vi "microFPGA_laser_sequence_addr_20_ctrl.vi"(0 "VISA resource name":refnum<visa-resource-name>, 1 "laser channel":u16(ring)=3 items=["channel No 0", "channel No 1", "channel No 2", "channel No 3", "channel No 4", "channel No 5", "channel No 6"], 2 "write or read":u16(ring) items=["read", "write"], 5 "sequence write":bool[](array[boolean])=[FALSE, FALSE, FALSE, FALSE, FALSE, FALSE, FALSE, FALSE, FALSE, FALSE, FALSE, FALSE, FALSE, FALSE, FALSE, FALSE], 11 "error in (no error)":errorcluster) -> (4 "VISA resource name 2":refnum<visa-resource-name>, 6 "sequence read":bool[](array[boolean]), 8 "value write confirm":bool, 10 "abort_wrong_input":bool, 15 "error out":errorcluster)   [LabVIEW 2016]
panel:
  out "mode read string answer":string
  out "mode read string":string
  out "mode write string":string
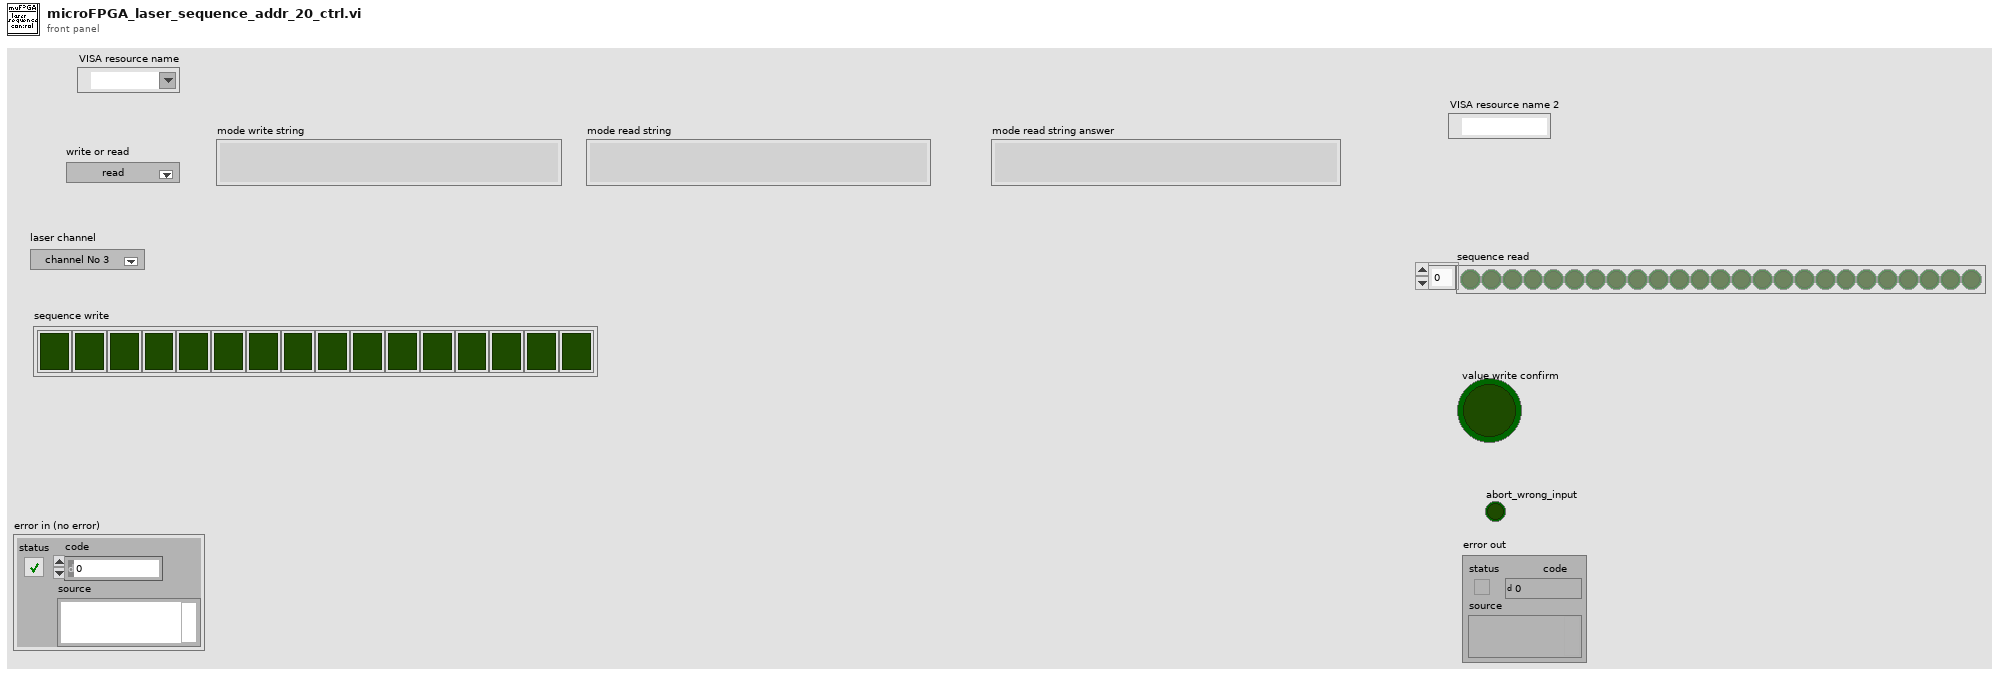
[diagram p1: front panel]
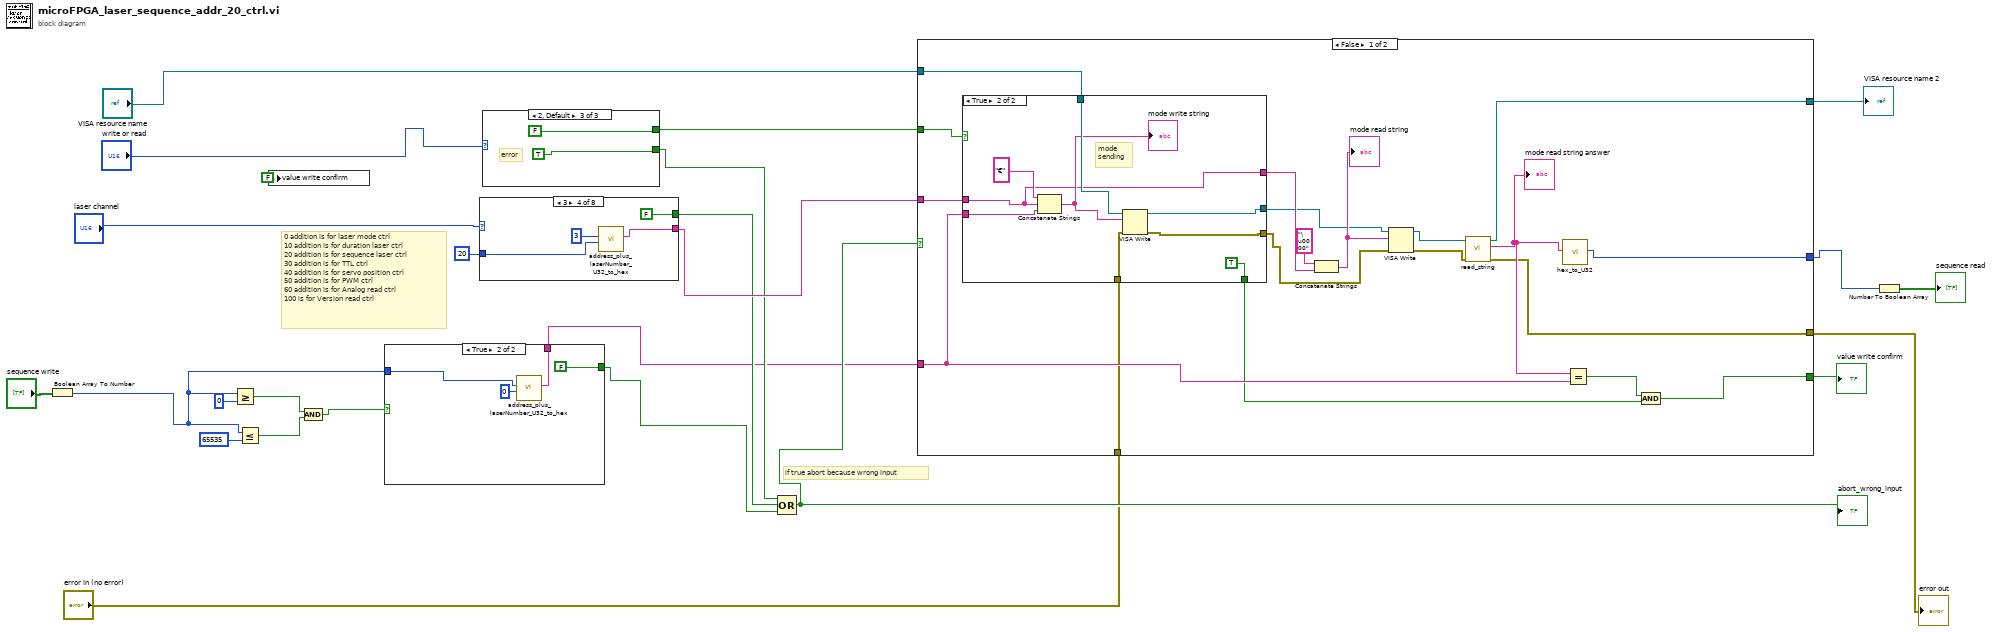
[diagram p0: block diagram]
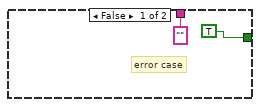
[diagram p2: hidden frame]
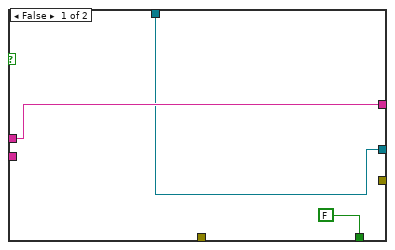
[diagram p3: hidden frame]
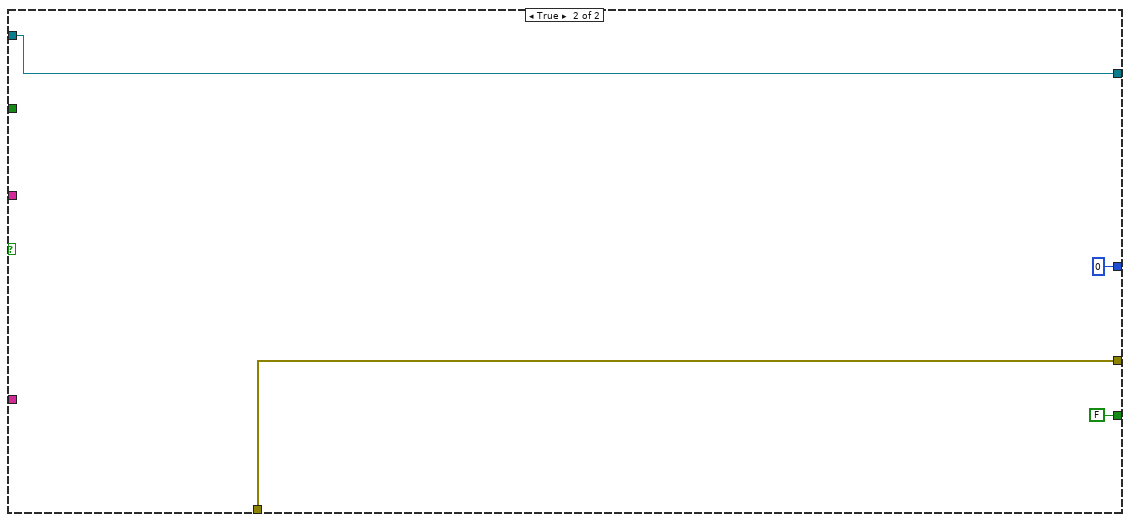
[diagram p4: hidden frame]
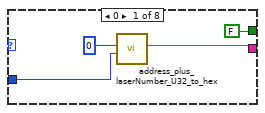
[diagram p5: hidden frame]
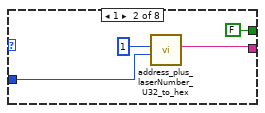
[diagram p6: hidden frame]
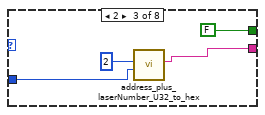
[diagram p7: hidden frame]
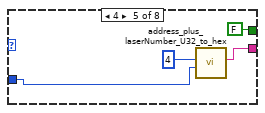
[diagram p8: hidden frame]
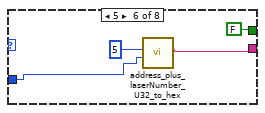
[diagram p9: hidden frame]
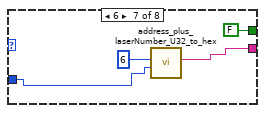
[diagram p10: hidden frame]
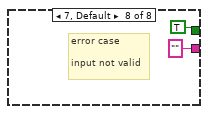
[diagram p11: hidden frame]
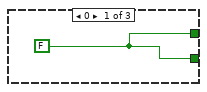
[diagram p12: hidden frame]
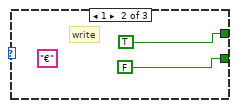
[diagram p13: hidden frame]
diagram:
  # "0 addition is for laser mode ctrl\n10 addition is for duration laser ctrl\n20 addition is for sequence laser ctrl\n30 addition is for TTL ctrl\n40 addition is for servo position ctrl\n50 addition is for PWM ctrl\n60 addition is for Analog read ctrl\n100 is for Version read ctrl"
  # "if true abort because wrong input"
  n1 = Boolean Array To Number(Boolean array="sequence write") -> (number=w4:u32)
  n2 = Greater Or Equal?(x=w4, y=u32 0) -> (x >= y?=w10:bool)
  n3 = Less Or Equal?(x=w4, y=u32 65535) -> (x <= y?=w9:bool)
  n4 = local write "value write confirm"(FALSE ("value confirm")) -> ()
  n5 = And(x=w10, y=w9) -> (x .and. y?=w8:bool)
  n6 = case shown="True" w8 {
    tunnel: w4 -> [_ w30]
    tunnel: [TRUE FALSE] -> w7
    tunnel: ["" ("string 5") w28] -> w6
    frame False {
      # "error case"
    }
    frame True {
      n7 = call "address_plus_laserNumber_U32_to_hex.vi"("adress offset"=u32 0, "y 3"=w30) -> ("string 5"=w28:string)  [unwired: 8 in]
    }
  }
  n8 = case shown="3" "laser channel" {
    tunnel: [w33 w37 w41 w45 w49 w53 w57 "" ("string 5")] -> w23
    tunnel: [FALSE FALSE FALSE FALSE FALSE FALSE FALSE TRUE] -> w19
    tunnel: u32 20 ("adress offset") -> [w32 w36 w40 w44 w48 w52 w56 _]
    frame 0 {
      n9 = call "address_plus_laserNumber_U32_to_hex.vi"("adress offset"=w32, "y 3"=u32 0) -> ("string 5"=w33:string)  [unwired: 8 in]
    }
    frame 1 {
      n10 = call "address_plus_laserNumber_U32_to_hex.vi"("adress offset"=w36, "y 3"=u32 1) -> ("string 5"=w37:string)  [unwired: 8 in]
    }
    frame 2 {
      n11 = call "address_plus_laserNumber_U32_to_hex.vi"("adress offset"=w40, "y 3"=u32 2) -> ("string 5"=w41:string)  [unwired: 8 in]
    }
    frame 3 {
      n12 = call "address_plus_laserNumber_U32_to_hex.vi"("adress offset"=w44, "y 3"=u32 3) -> ("string 5"=w45:string)  [unwired: 8 in]
    }
    frame 4 {
      n13 = call "address_plus_laserNumber_U32_to_hex.vi"("adress offset"=w48, "y 3"=u32 4) -> ("string 5"=w49:string)  [unwired: 8 in]
    }
    frame 5 {
      n14 = call "address_plus_laserNumber_U32_to_hex.vi"("adress offset"=w52, "y 3"=u32 5) -> ("string 5"=w53:string)  [unwired: 8 in]
    }
    frame 6 {
      n15 = call "address_plus_laserNumber_U32_to_hex.vi"("adress offset"=w56, "y 3"=u32 6) -> ("string 5"=w57:string)  [unwired: 8 in]
    }
    frame 7, Default {
      # "error case\n\ninput not valid"
    }
  }
  n16 = case shown="2, Default" "write or read" {
    tunnel: [w62 TRUE FALSE] -> w22
    tunnel: [w62 FALSE TRUE] -> w20
    frame 0 {
      w62 = FALSE
    }
    frame 1 {
      (unwired) "€" ("hex")
      # "write"
    }
    frame 2, Default {
      # "error"
    }
  }
  n17 = Compound Arithmetic op=OR(w20, w19, w7) -> (w17:bool)
  "abort_wrong_input" <- w17
  n18 = case shown="False" w17 {
    tunnel: "VISA resource name" -> [w85 w99]
    tunnel: w23 -> [w82 _]
    tunnel: w22 -> [w76 _]
    tunnel: w6 -> [w74 _]
    tunnel: [w73 u32 0 ("U32")] -> w2
    tunnel: [w67 FALSE] -> w18
    tunnel: [w72 w99] -> w16
    tunnel: "error in (no error)" -> [w71 w98]
    tunnel: [w70 w98] -> w14
    frame False {
      n19 = case shown="True" w76 {
        tunnel: w82 -> [w88 w94]
        tunnel: w85 -> [w87 w96]
        tunnel: [w88 w94] -> w83
        tunnel: w74 -> [_ w93]
        tunnel: [w87 w92] -> w78
        tunnel: [_ w91] -> w77
        tunnel: w71 -> [_ w90]
        tunnel: [FALSE TRUE] -> w69
        frame False {
        }
        frame True {
          # "mode \nsending"
          n20 = Concatenate Strings("€" ("string"), w94, w93) -> (w95:string)
          "mode write string" <- w95
          n21 = VISA Write(VISA resource name=w96, write buffer=w95, error in (no error)=w90) -> (VISA resource name out=w92:refnum<visa-resource-name>, error out=w91:errorcluster)  [unwired: 1 out]
        }
      }
      n22 = Concatenate Strings("\u0000" ("string"), w83) -> (w81:string)
      "mode read string" <- w81
      n23 = VISA Write(VISA resource name=w78, write buffer=w81, error in (no error)=w77) -> (VISA resource name out=w80:refnum<visa-resource-name>, error out=w79:errorcluster)  [unwired: 1 out]
      n24 = call "read_string.vi"("error in"=w79, "VISA resource name"=w80) -> ("error out"=w70:errorcluster, "read buffer"=w75:string, "VISA resource name out"=w72:refnum<visa-resource-name>)  [unwired: 7 in]
      "mode read string answer" <- w75
      n25 = call "hex_to_U32.vi"("hex"=w75) -> ("U32"=w73:u32)  [unwired: 9 in]
      n26 = Equal?(x=w75, y=w74) -> (x = y?=w68:bool)
      n27 = And(x=w68, y=w69) -> (x .and. y?=w67:bool)
    }
    frame True {
    }
  }
  "value write confirm" <- w18
  "VISA resource name 2" <- w16
  "error out" <- w14
  n28 = Number To Boolean Array(number=w2) -> (Boolean array=→"sequence read":bool[])
